vi "ErrorLogString.vi"(8 "错误输入":errorcluster) -> (0 "错误输出":errorcluster, 3 "LogString":string)   [LabVIEW 2018, in "ErrorHanlder.lvlib" / "ErrorHanlder.lvclass"]
uses:
  ErrorHanlder.lvclass
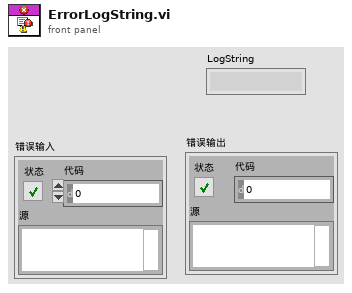
[diagram p1: front panel]
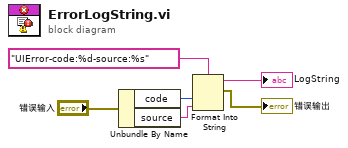
[diagram p0: block diagram]
diagram:
  n1 = Unbundle By Name("错误输入") -> ("code"=w3:i32, "source"=w2:string)
  n2 = Format Into String(format string="UIError-code:%d-source:%s" ("格式字符串"), w3, w2) -> (resulting string=→"LogString":string, error out=→"错误输出":errorcluster)  [unwired: 2 in]
